vi "Search.vi"() -> ()   [LabVIEW 2021]
uses:
  System.Windows.Forms
panel:
  in  "Search":bool
  in  "SEARCH":string
  in  "Combo Box":string(combo)
  in  "Google":bool
  in  "WebBrowser":refnum<k24>(container)
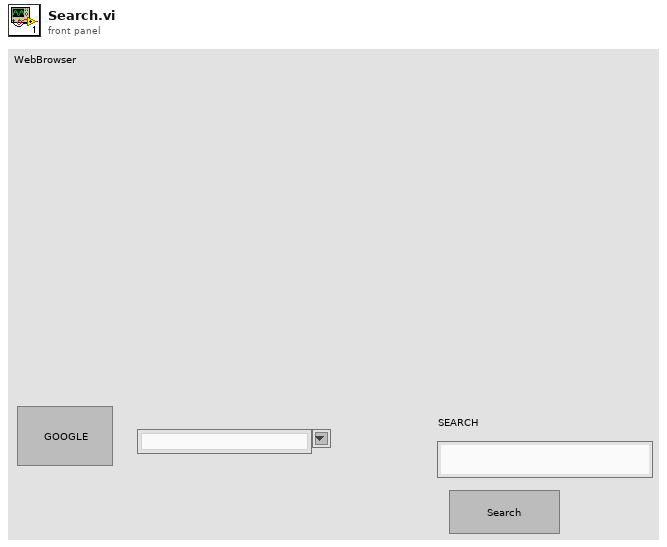
[diagram p1: front panel]
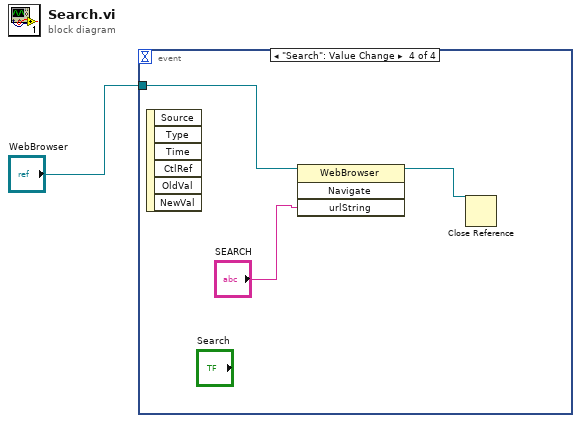
[diagram p0: block diagram]
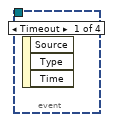
[diagram p2: hidden frame]
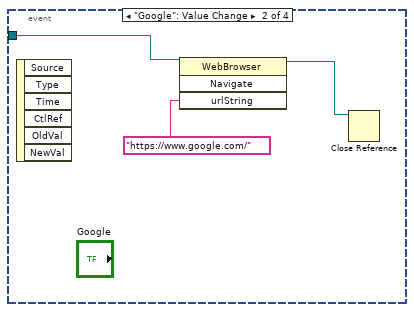
[diagram p3: hidden frame]
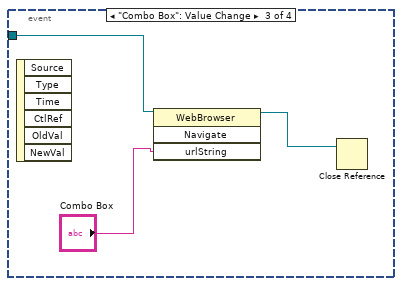
[diagram p4: hidden frame]
diagram:
  n1 = event shown="[3] \"Search\": Value Change" {
    selector: _ -> [_ _ _ _]
    dyn-events: _ -> [_ _ _ _]
    timeout: _ -> [_ _ _ _]
    tunnel: "WebBrowser" -> [_ w3 w6 w9]
    event Timeout {
      n2 = event-data() -> ()  [unwired: 1 in, 3 out]
    }
    event "Google": Value Change {
      n3 = event-data() -> ()  [unwired: 1 in, 6 out]
      n4 = invoke class="WebBrowser" method="Navigate"(reference=w3, "urlString"="https://www.google.com/") -> (reference out=w2:refnum<k24>)  [unwired: 2 in, 3 out]
      n5 = Close Reference(reference=w2) -> ()  [unwired: 1 in, 1 out]
    }
    event "Combo Box": Value Change {
      n6 = event-data() -> ()  [unwired: 1 in, 6 out]
      n7 = invoke class="WebBrowser" method="Navigate"(reference=w6, "urlString"="Combo Box") -> (reference out=w5:refnum<k24>)  [unwired: 2 in, 3 out]
      n8 = Close Reference(reference=w5) -> ()  [unwired: 1 in, 1 out]
    }
    event "Search": Value Change {
      n9 = event-data() -> ()  [unwired: 1 in, 6 out]
      n10 = invoke class="WebBrowser" method="Navigate"(reference=w9, "urlString"="SEARCH") -> (reference out=w8:refnum<k24>)  [unwired: 2 in, 3 out]
      n11 = Close Reference(reference=w8) -> ()  [unwired: 1 in, 1 out]
    }
  }
